vi "Launch Cylinder.vi"(8 "error in (no error)":errorcluster, 11 "cRIO-CO2 in":refnum<class "cRIO-CO2.lvclass">) -> (0 "error out":errorcluster, 3 "cRIO-CO2 out":refnum<class "cRIO-CO2.lvclass">)   [LabVIEW 2015, in "cRIO-Carbondioxide.lvlib" / "cRIO-CO2.lvlib" / "cRIO-CO2.lvclass"]
uses:
  cRIO-CO2.lvclass
  <vilib>/ActorFramework/Actor/Actor.lvclass
  cRIO-CO2.lvclass/cRIO-CO2.ctl
  cRIO-CO2 Messages/Log Message Msg/Log Message Msg.lvclass/Log Message Msg.ctl
  <vilib>/ActorFramework/Message Enqueuer/Message Enqueuer.lvclass/Message Enqueuer.ctl
  <vilib>/ActorFramework/Message Enqueuer/Enqueue.vi
  <vilib>/ActorFramework/Message Priority Queue/Priority Enqueue.vi
  cRIO-CO2 Messages/Log Message Msg/Log Message Msg.lvclass
  <vilib>/ActorFramework/Message Enqueuer/Message Enqueuer.lvclass
  Cylinder/Cylinder.lvclass
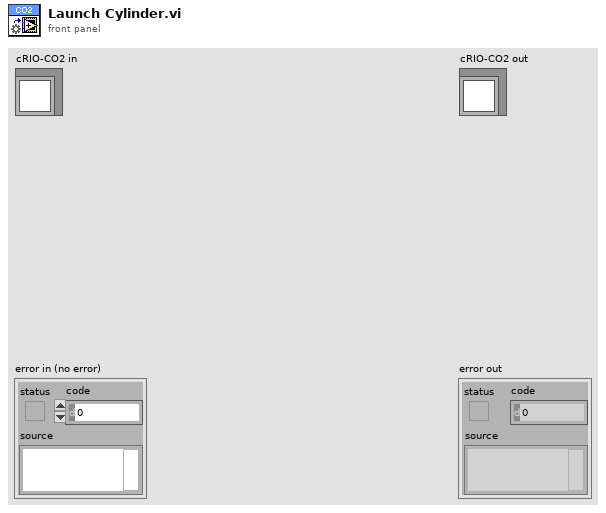
[diagram p1: front panel]
types:
  T1 = cluster{"Pressure Setpoint Control ":refnum<k21>, "Analog output":refnum<k21>, "Direction Valve IO":refnum<k21>, "Home Control":refnum<k21>, "Position Sensor":refnum<k21>}
  T2 = typedef "Dedicated Enqueuers.ctl" = cluster{"Freezers":cluster{"Syringe":refnum<class "Message Enqueuer.lvclass">, "Tank 1":refnum<class "Message Enqueuer.lvclass">, "Tank 2":refnum<class "Message Enqueuer.lvclass">, "Tank 3":refnum<class "Message Enqueuer.lvclass">, "Tank 4":refnum<class "Message Enqueuer.lvclass">}, "Heaters":cluster{"Syringe":refnum<class "Message Enqueuer.lvclass">, "Piston":refnum<class "Message Enqueuer.lvclass">}, "Blowers":cluster{"Tank 1":refnum<class "Message Enqueuer.lvclass">, "Tank 2":refnum<class "Message Enqueuer.lvclass">, "Tank 3":refnum<class "Message Enqueuer.lvclass">, "Tank 4":refnum<class "Message Enqueuer.lvclass">, "Syringe":refnum<class "Message Enqueuer.lvclass">}, "Sample Line":refnum<class "Message Enqueuer.lvclass">, "Storage Line":refnum<class "Message Enqueuer.lvclass">, "Transfer Line":refnum<class "Message Enqueuer.lvclass">, "Syringe Stepper":refnum<class "Message Enqueuer.lvclass">, "Syringe Line":refnum<class "Message Enqueuer.lvclass">, "Capillary Line":refnum<class "Message Enqueuer.lvclass">, "Preparation Line":refnum<class "Message Enqueuer.lvclass">, "Turbo":refnum<class "Message Enqueuer.lvclass">, "Vacuum":refnum<class "Message Enqueuer.lvclass">, "He Line":refnum<class "Message Enqueuer.lvclass">, "Cylinder":refnum<class "Message Enqueuer.lvclass">}
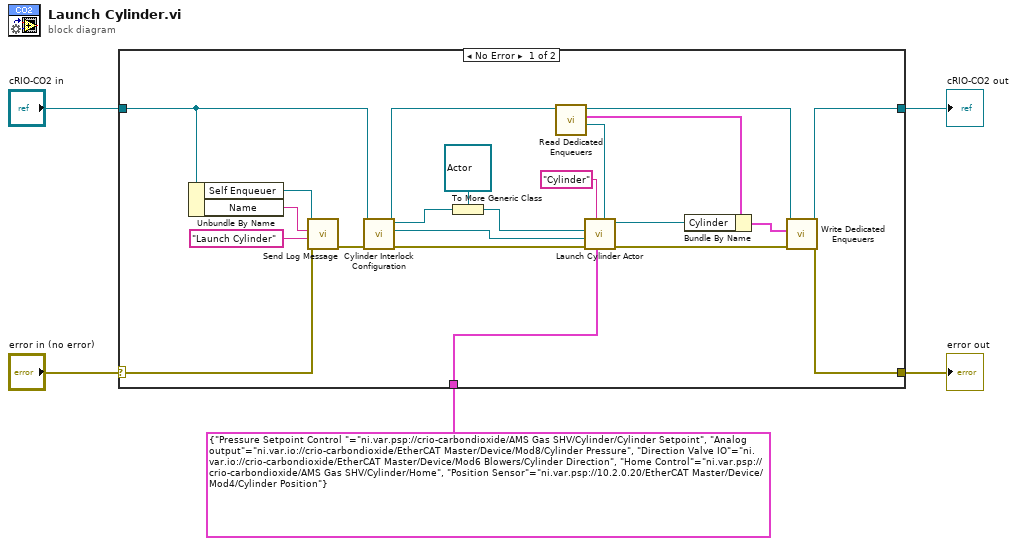
[diagram p0: block diagram]
diagram:
  n1 = case shown="No Error" "error in (no error)" {
    selector: "error in (no error)" -> [w24 w28]
    tunnel: [w14 w28] -> w4
    tunnel: [w18 w27] -> w2
    tunnel: "cRIO-CO2 in" -> [w21 w27]
    tunnel: T1 {"Pressure Setpoint Control "="ni.var.psp://crio-carbondioxide/AMS Gas SHV/Cylinder/Cylinder Setpoint", "Analog output"="ni.var.io://crio-carbondioxide/EtherCAT Master/Device/Mod8/Cylinder Pressure", "Direction Valve IO"="ni.var.io://crio-carbondioxide/EtherCAT Master/Device/Mod6 Blowers/Cylinder Direction", "Home Control"="ni.var.psp://crio-carbondioxide/AMS Gas SHV/Cylinder/Home", "Position Sensor"="ni.var.psp://10.2.0.20/EtherCAT Master/Device/Mod4/Cylinder Position"} ("SHVs") -> [w6 _]
    frame No Error {
      n2 = Unbundle By Name(w21) -> ("Self Enqueuer"=w23:refnum<class "Message Enqueuer.lvclass">, "Name"=w26:string)
      n3 = call "Send Log Message.vi"("error in (no error)"=w24, "String"="Launch Cylinder", "Source Name"=w26, "Message Enqueuer"=w23) -> ("error out"=w22:errorcluster)  [unwired: 6 in, 1 out]
      n4 = call "Cylinder Interlock Configuration.vi"("error in (no error)"=w22, "cRIO-CO2 in"=w21) -> ("error out"=w20:errorcluster, "Interlock Chain"=w19:refnum<class "Interlock Chain.lvclass">, "cRIO-CO2 out"=w8:refnum<class "cRIO-CO2.lvclass">)  [unwired: 7 in]
      n5 = To More Generic Class(target class=refnum<class "Actor.lvclass"> refnum ("Caller Actor in"), reference=w8) -> (generic class reference=w7:refnum<class "Actor.lvclass">)
      n6 = call "Read Dedicated Enqueuers.vi"("cRIO-CO2 in"=w8) -> ("Qs.DedicatedEnQrs"=w10:refnum<queue>, "Dedicated Enqueuers"=w17:T2, "cRIO-CO2 out"=w9:refnum<class "cRIO-CO2.lvclass">)  [unwired: 7 in, 1 out]
      n7 = call "Launch Cylinder Actor.vi"("DedicatedEnQrs"=w10, "SHVs"=w6, "Name"="Cylinder", "error in (no error)"=w20, "Interlock Chain"=w19, "Caller Actor in"=w7) -> ("error out"=w11:errorcluster, "Caller-To-Actor Enqueuer"=w15:refnum<class "Message Enqueuer.lvclass">)  [unwired: 4 in]
      n8 = Bundle By Name(cluster=w17, "Cylinder"=w15) -> (w16:T2)
      n9 = call "Write Dedicated Enqueuers.vi"("error in (no error)"=w11, "Dedicated Enqueuers"=w16, "cRIO-CO2 in"=w9) -> ("error out"=w14:errorcluster, "cRIO-CO2 out"=w18:refnum<class "cRIO-CO2.lvclass">)  [unwired: 7 in]
    }
    frame Error {
    }
  }
  "error out" <- w4
  "cRIO-CO2 out" <- w2
